vi "patientTrashtListView.vi"() -> ()   [LabVIEW 2019]
uses:
  03_Home/controller/logoutBtn.ctl
  03_Home/controller/exitBtn.ctl
  <vilib>/Utility/miscctls.llb/LVPointTypeDef.ctl
  subVI/patients_state.ctl
  03_Home/controller/pannelState.ctl
  globalValue.vi
panel:
  in  "btnGroup":T1
  in  "backPage":bool
  out "x-y*floor(x/y)":i32
  out "totalCount":string
  out "totalPage":i8
  out "crrentPage":i8
  in  "leftBtn":bool
  in  "rightBtn":bool
  out "patientList":i32(listbox)
  in  "searchBtn":bool
  in  "searchForm":string
  in  "Help Button":bool
  in  "LogOut Button":T2
  in  "Exit Button":T3
  out "userNm":string
  # "/"
  # "|"
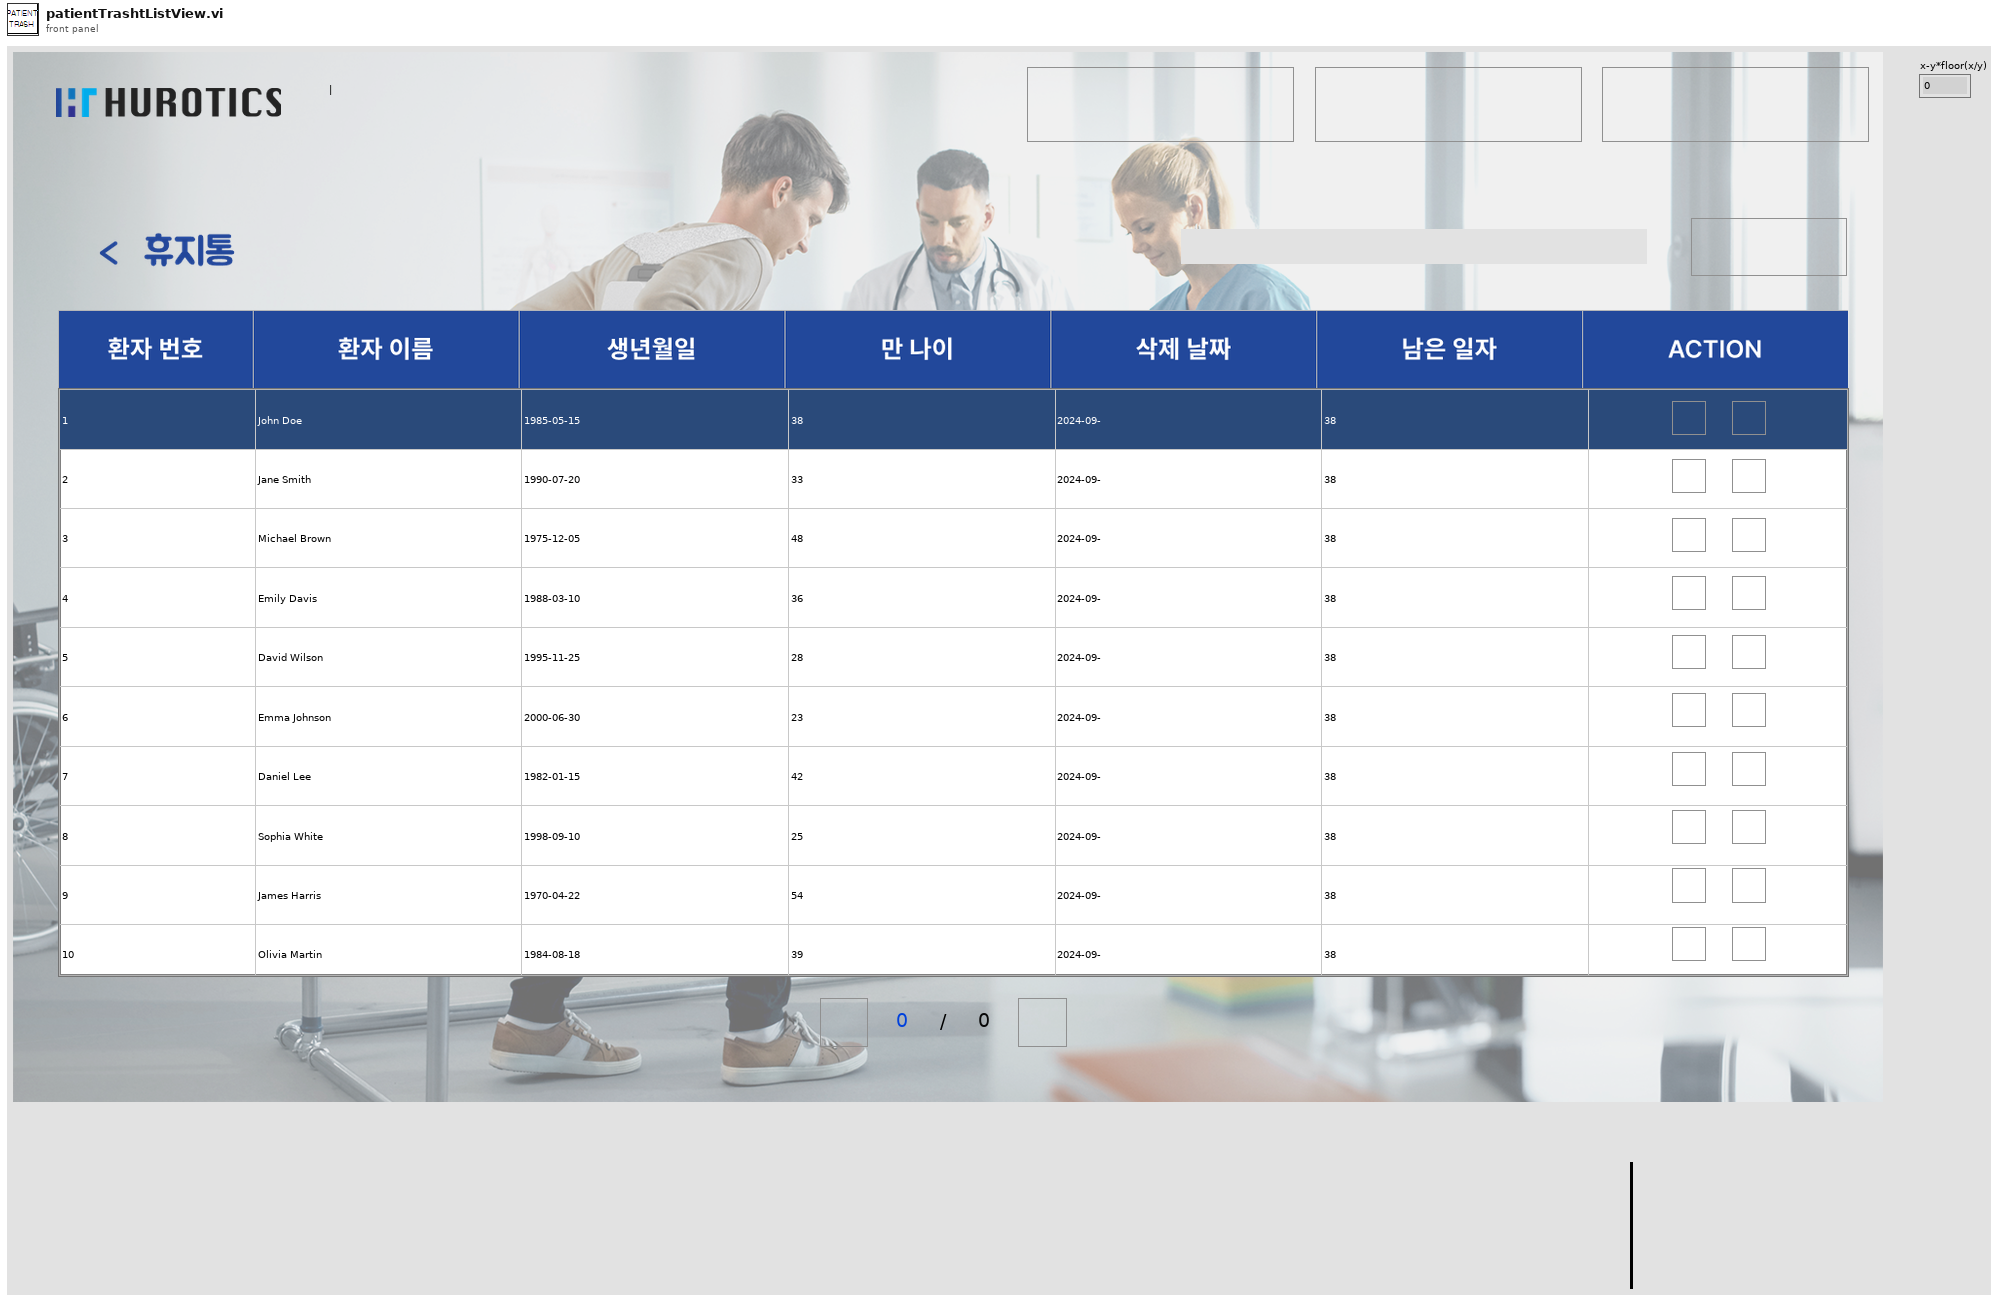
[diagram p1: front panel]
types:
  T1 = cluster{"updateBtn":bool, "deleteBtn":bool, "updateBtn 2":bool, "deleteBtn 2":bool, "updateBtn 3":bool, "deleteBtn 3":bool, "updateBtn 4":bool, "deleteBtn 4":bool, "updateBtn 5":bool, "deleteBtn 5":bool, "updateBtn 6":bool, "deleteBtn 6":bool, "updateBtn 7":bool, "deleteBtn 7":bool, "updateBtn 8":bool, "deleteBtn 8":bool, "updateBtn 9":bool, "deleteBtn 9":bool, "updateBtn 10":bool, "deleteBtn 10":bool}
  T2 = typedef "logoutBtn.ctl" = bool
  T3 = typedef "exitBtn.ctl" = bool
  T4 = typedef "LVPointTypeDef.ctl" = cluster{"Horizontal":i16, "Vertical":i16}
  T5 = enum16{"connection", "create", "getReadList", "getRead", "getCount", "update", "delete", "close"}
  T6 = typedef "patients_state.ctl" = enum16{"connection", "create", "getReadList", "getRead", "getCount", "update", "delete", "trash", "restore", "close"}
  T7 = enum8{"Enabled", "Disabled", "Disabled and Grayed Out"}
  T8 = typedef "pannelState.ctl" = enum16{"Init", "LogIn", "SignUpView", "Home", "Management_patientList", "Management_patientTrashtList", "Management_patientCreate", "Management_patientUpdate", "Management_patientTraining", "Management_patientTrainingDetail", "H-MEDI PatientList", "H-MEDI HardwareCtl", "Adjust", "FineTuning", "UserList", "UserDetail", "Exit"}
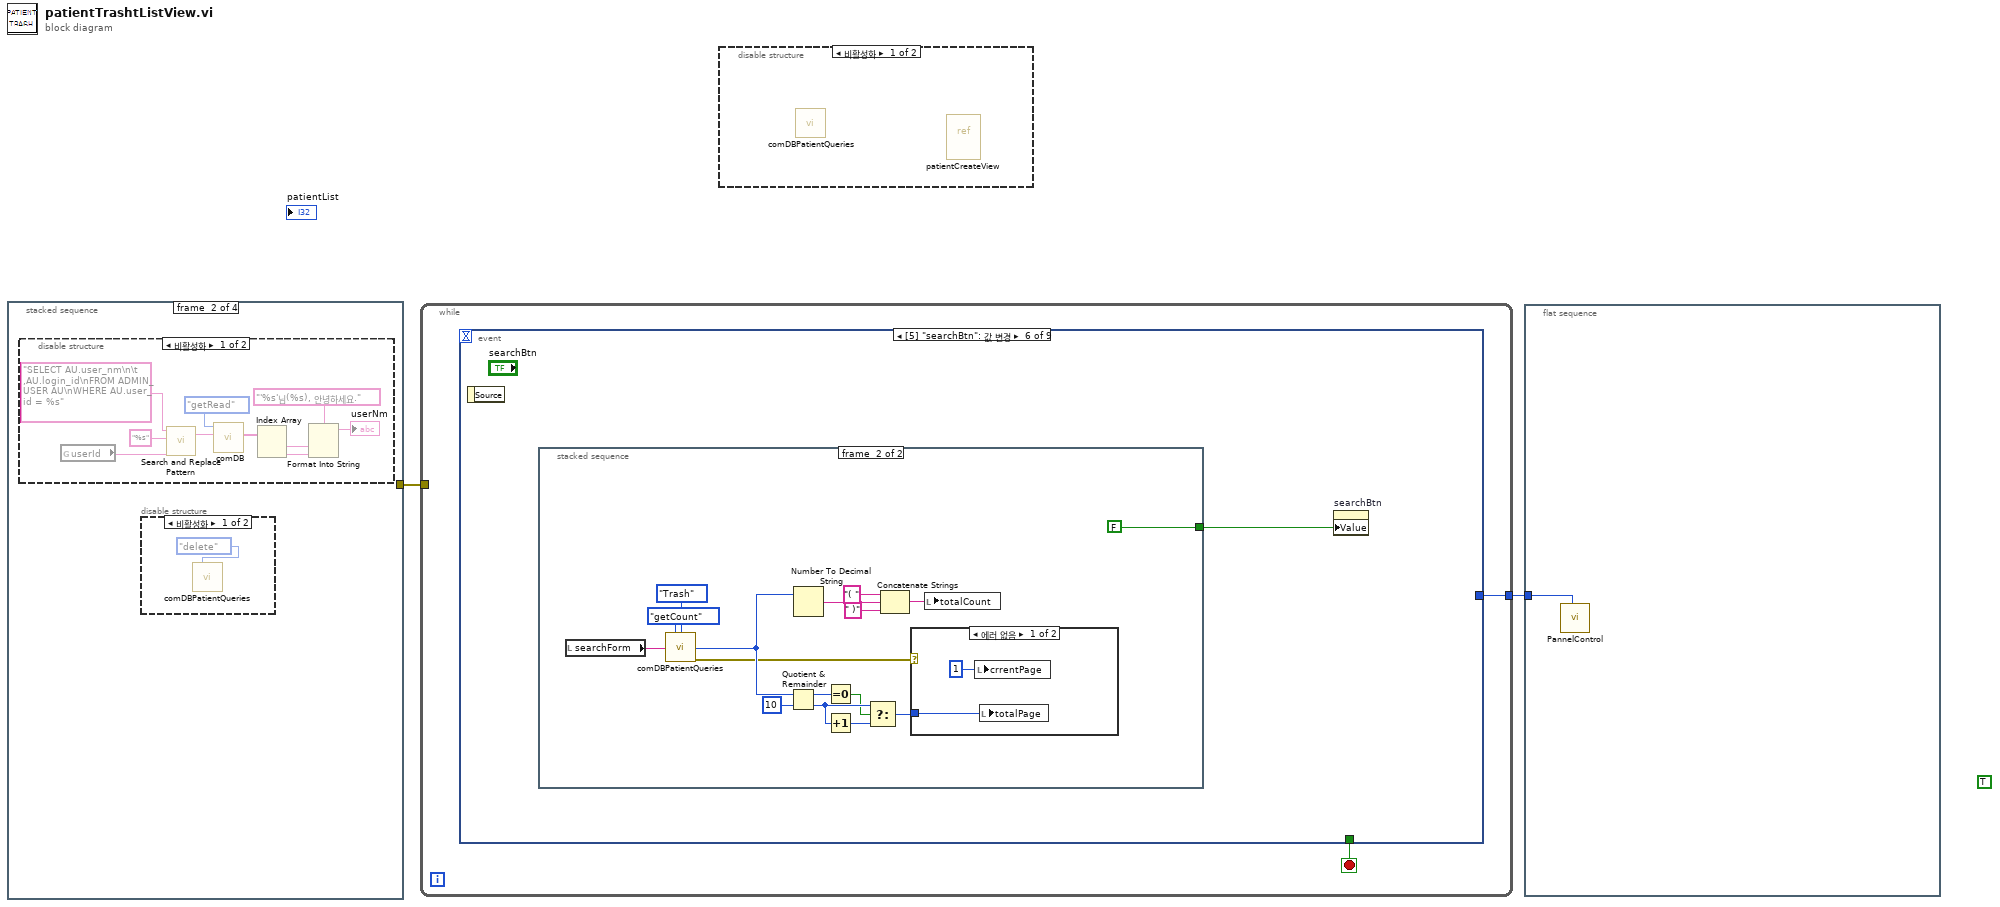
[diagram p0: block diagram]
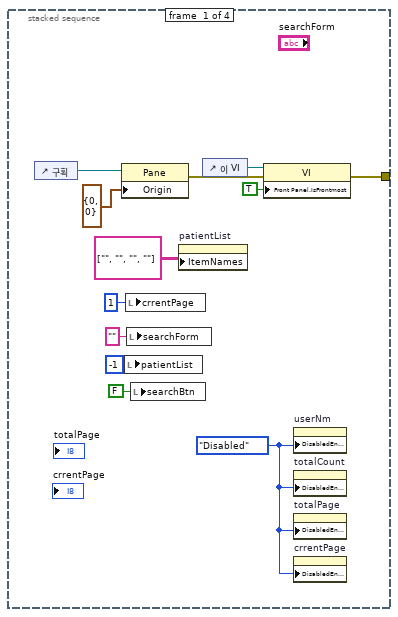
[diagram p3: hidden frame]
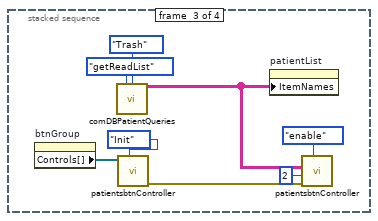
[diagram p6: hidden frame]
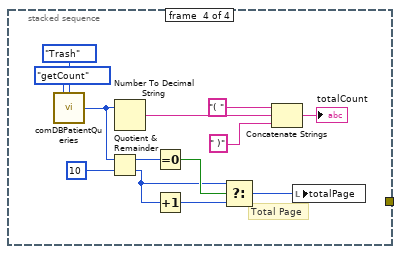
[diagram p7: hidden frame]
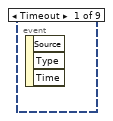
[diagram p8: hidden frame]
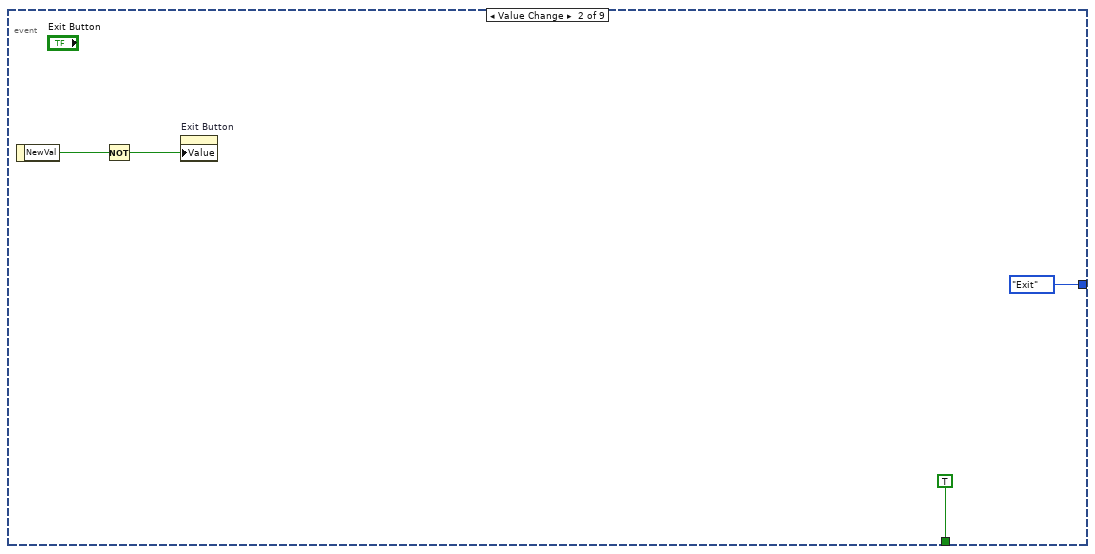
[diagram p9: hidden frame]
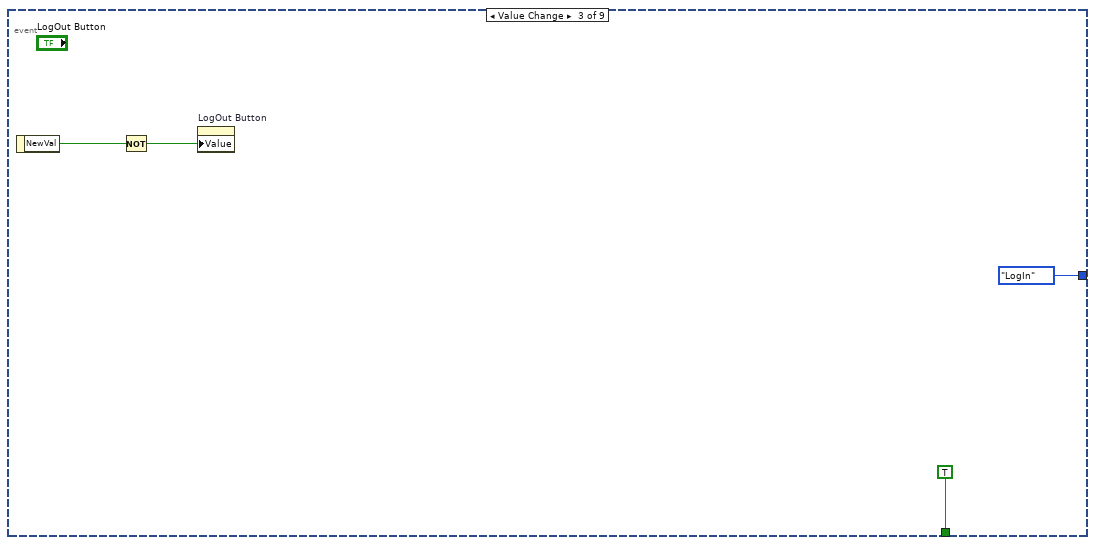
[diagram p10: hidden frame]
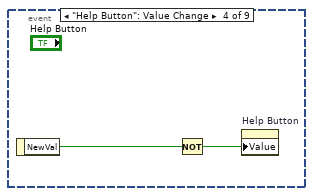
[diagram p11: hidden frame]
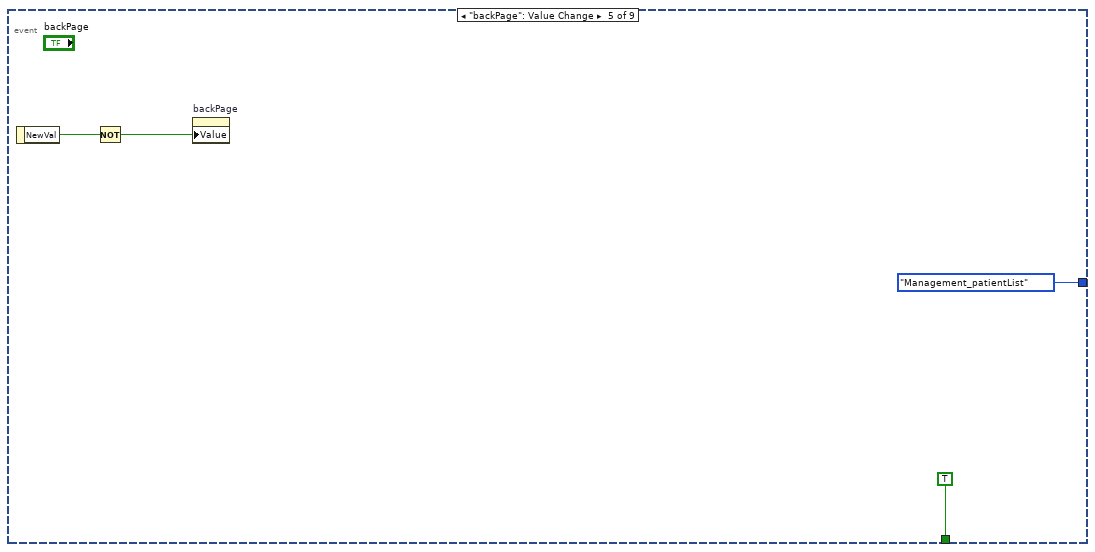
[diagram p12: hidden frame]
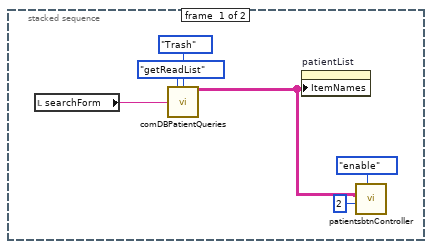
[diagram p13: hidden frame]
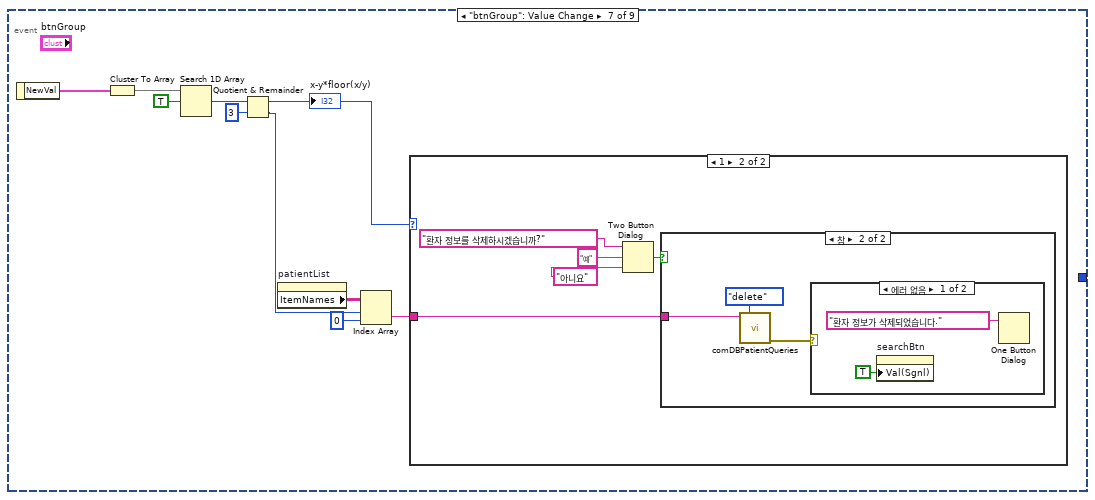
[diagram p15: hidden frame]
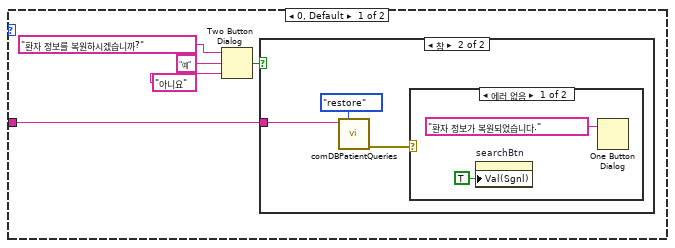
[diagram p16: hidden frame]
diagram:
  (unwired) TRUE
  n1 = stacked-sequence {
    tunnel: [w5 _ _ _] -> w2
    frame #0 {
      w4 = T7."Disabled" ("비활성화")
      n2 = control-ref of="구획"() -> (w12:refnum<vi>)
      n3 = property class="Pane"(reference=w12, "Origin"=T4 {"Horizontal"=0, "Vertical"=0} ("원점")) -> (error out=w10:errorcluster)  [unwired: 1 in, 1 out]
      n4 = local write "patientList"(-1 ("userList")) -> ()
      n5 = local write "crrentPage"(i8 1 ("crrentPage")) -> ()
      n6 = local write "searchForm"("" ("searchForm")) -> ()
      n7 = local write "searchBtn"(FALSE ("searchBtn")) -> ()
      n8 = property on="patientList" class="MCListbox (엄격한)"("ItemNames"=string[][] [["", ""], ["", ""]]) -> ()  [unwired: 2 in, 2 out]
      n9 = control-ref of="이 VI"() -> (w14:refnum<vi>)
      n10 = property class="VI"(reference=w14, error in=w10, "Front Panel.IsFrontmost"=TRUE ("프런트패널 윈도우:맨 앞으로")) -> (error out=w5:errorcluster)  [unwired: 1 out]
      n11 = property on="userNm" class="Str"("DisabledEnum"=w4) -> ()  [unwired: 2 in, 2 out]
      n12 = property on="totalCount" class="Str"("DisabledEnum"=w4) -> ()  [unwired: 2 in, 2 out]
      n13 = property on="totalPage" class="DigNum (엄격한)"("DisabledEnum"=w4) -> ()  [unwired: 2 in, 2 out]
      n14 = property on="crrentPage" class="DigNum (엄격한)"("DisabledEnum"=w4) -> ()  [unwired: 2 in, 2 out]
    }
    frame #1 {
      n15 = disable-structure shown="비활성화" {
        frame Disabled {
          n16 = global read "globalValue.vi" "userId"() -> (w15:string)
          n17 = call <vilib>:"Search and Replace Pattern.vi"("string"="SELECT AU.user_nm\n\t         ,AU.login_id\nFROM ADMIN_USER AU\nWHERE AU.user_id = %s" ("Query"), "regular expression (\"\")"="%s" ("regular expression (\"\")"), "replace string (\"\")"=w15) -> ("result string"=w17:string)  [unwired: 2 in, 1 out]
          n18 = call "comDB.vi"("Query"=w17, "State"=T5."getRead") -> ("result1DArray"=w22:string[])  [unwired: 5 in, 3 out]
          n19 = Index Array(array=w22) -> (element #1=w21:string, element #2=w20:string)  [unwired: 2 in]
          n20 = Format Into String(format string="'%s'님(%s), 안녕하세요." ("문자열"), w21, w20) -> (resulting string=→"userNm":string)  [unwired: 2 in, 1 out]
        }
        frame Enabled {
        }
      }
      n21 = disable-structure shown="비활성화" {
        frame Disabled {
          n22 = call "comDBPatientQueries.vi"("State"=patients_state."delete") -> ()  [unwired: 11 in, 4 out]
        }
        frame Enabled {
        }
      }
    }
    frame #2 {
      n23 = property on="btnGroup" class="Clust"() -> ("Controls[]"=w27:refnum<vi>[])  [unwired: 2 in, 2 out]
      n24 = call "comDBPatientQueries.vi"("State"=patients_state."getReadList", "select"=enum16{"Default", "Trash", "Training"}."Trash") -> ("resultList"=w29:string[][])  [unwired: 10 in, 3 out]
      n25 = call "patientsbtnController.vi"("state"=enum16{"Init", "disable", "enable"}."Init", "Controls[]"=w27) -> ("error out"=w30:errorcluster)  [unwired: 9 in]
      n26 = property on="patientList" class="MCListbox (엄격한)"("ItemNames"=w29) -> ()  [unwired: 2 in, 2 out]
      n27 = call "patientsbtnController.vi"("state"=enum16{"Init", "disable", "enable"}."enable", "error in (no error)"=w30, "버튼개수"=2, "2dArray"=w29) -> ()  [unwired: 7 in, 1 out]
    }
    frame #3 {
      # "Total Page"
      n28 = call "comDBPatientQueries.vi"("State"=patients_state."getCount", "select"=enum16{"Default", "Trash", "Training"}."Trash") -> ("count"=w35:i64)  [unwired: 10 in, 3 out]
      n29 = Quotient & Remainder(x=w35, y=i64 10) -> (x-y*floor(x/y)=w38:i64, floor(x/y)=w37:i64)
      n30 = Number To Decimal String(number=w35) -> (decimal integer string=w44:string)  [unwired: 1 in]
      n31 = Equal To 0?(x=w38) -> (x = 0?=w39:bool)
      n32 = Increment(x=w37) -> (x+1=w41:i64)
      n33 = Select(t=w37, s=w39, f=w41) -> (s? t:f=w40:i64)
      n34 = Concatenate Strings("( ", w44, " )") -> (→"totalCount":string)
      n35 = local write "totalPage"(w40) -> ()
    }
  }
  n36 = while {
    tunnel: w2 -> [_]
    tunnel: [w47] -> w1
    stop <- w48 stop-if-true
    n37 = event shown="[5] \"searchBtn\": 값 변경" {
      selector: _ -> [_ _ _ _ _ _ _ _ _]
      dyn-events: _ -> [_ _ _ _ _ _ _ _ _]
      timeout: _ -> [_ _ _ _ _ _ _ _ _]
      tunnel: [_ TRUE TRUE _ TRUE _ _ _ _] -> w48
      tunnel: [_ pannelState."Exit" ("State") pannelState."LogIn" ("State") _ pannelState."Management_patientList" ("State") _ _ _ _] -> w47
      event Timeout {
        n38 = event-data() -> ()  [unwired: 1 in, 3 out]
      }
      event Value Change {
        n39 = event-data() -> ("NewVal"=w50:T3)  [unwired: 1 in]
        n40 = Not(x=w50) -> (.not. x?=w49:T3)
        n41 = property on="Exit Button" class="Bool (엄격한)"("Value"=w49) -> ()  [unwired: 2 in, 2 out]
      }
      event Value Change {
        n42 = event-data() -> ("NewVal"=w56:T2)  [unwired: 1 in]
        n43 = Not(x=w56) -> (.not. x?=w55:T2)
        n44 = property on="LogOut Button" class="Bool (엄격한)"("Value"=w55) -> ()  [unwired: 2 in, 2 out]
      }
      event "Help Button": Value Change {
        n45 = event-data() -> ("NewVal"=w58:bool)  [unwired: 1 in]
        n46 = Not(x=w58) -> (.not. x?=w57:bool)
        n47 = property on="Help Button" class="Bool (엄격한)"("Value"=w57) -> ()  [unwired: 2 in, 2 out]
      }
      event "backPage": Value Change {
        n48 = event-data() -> ("NewVal"=w60:bool)  [unwired: 1 in]
        n49 = Not(x=w60) -> (.not. x?=w59:bool)
        n50 = property on="backPage" class="Bool (엄격한)"("Value"=w59) -> ()  [unwired: 2 in, 2 out]
      }
      event "searchBtn": Value Change {
        n51 = event-data() -> ()  [unwired: 1 in, 1 out]
        n52 = stacked-sequence {
          tunnel: [_ FALSE ("searchBtn")] -> w63
          frame #0 {
            n53 = local read "searchForm"() -> (w67:string)
            n54 = call "comDBPatientQueries.vi"("State"=patients_state."getReadList", "select"=enum16{"Default", "Trash", "Training"}."Trash", "searchForm"=w67) -> ("resultList"=w66:string[][])  [unwired: 9 in, 3 out]
            n55 = property on="patientList" class="MCListbox (엄격한)"("ItemNames"=w66) -> ()  [unwired: 2 in, 2 out]
            n56 = call "patientsbtnController.vi"("state"=enum16{"Init", "disable", "enable"}."enable", "버튼개수"=2, "2dArray"=w66) -> ()  [unwired: 8 in, 1 out]
          }
          frame #1 {
            n57 = local read "searchForm"() -> (w73:string)
            n58 = call "comDBPatientQueries.vi"("State"=patients_state."getCount", "select"=enum16{"Default", "Trash", "Training"}."Trash", "searchForm"=w73) -> ("count"=w72:i64, "error out"=w71:errorcluster)  [unwired: 9 in, 2 out]
            n59 = Quotient & Remainder(x=w72, y=i64 10) -> (x-y*floor(x/y)=w77:i64, floor(x/y)=w78:i64)
            n60 = Number To Decimal String(number=w72) -> (decimal integer string=w82:string)  [unwired: 1 in]
            n61 = Equal To 0?(x=w77) -> (x = 0?=w76:bool)
            n62 = Increment(x=w78) -> (x+1=w80:i64)
            n63 = Select(t=w78, s=w76, f=w80) -> (s? t:f=w79:i64)
            n64 = Concatenate Strings("( ", w82, " )") -> (w83:string)
            n65 = case shown="에러 없음" w71 {
              tunnel: w79 -> [w86 _]
              frame No Error {
                n66 = local write "crrentPage"(i8 1 ("crrentPage")) -> ()
                n67 = local write "totalPage"(w86) -> ()
              }
              frame Error {
              }
            }
            n68 = local write "totalCount"(w83) -> ()
          }
        }
        n69 = property on="searchBtn" class="Bool (엄격한)"("Value"=w63) -> ()  [unwired: 2 in, 2 out]
      }
      event "btnGroup": Value Change {
        n70 = event-data() -> ("NewVal"=w89:T1)  [unwired: 1 in]
        n71 = Cluster To Array(cluster=w89) -> (array=w97:bool[])
        n72 = Search 1D Array(1D array=w97, element=TRUE ("원소")) -> (index of element=w96:i32)  [unwired: 1 in]
        n73 = Quotient & Remainder(x=w96, y=3) -> (x-y*floor(x/y)=w90:i32, floor(x/y)=w91:i32)
        "x-y*floor(x/y)" <- w90
        n74 = property on="patientList" class="MCListbox (엄격한)"() -> ("ItemNames"=w94:string[][])  [unwired: 2 in, 2 out]
        n75 = Index Array(array=w94, index (row)=w91, index (col)=0 ("비활성화된 인덱스 (열)")) -> (element=w92:string)
        n76 = case shown="1" w90 {
          tunnel: w92 -> [w99 w109]
          frame 0, Default {
            n77 = Two Button Dialog(message="환자 정보를 복원하시겠습니까?" ("메시지"), 1:"아니요" ("거짓 버튼 이름(\"취소\")"), 2:"예" ("참 버튼 이름(\"확인\")")) -> (T button?=w98:bool)
            n78 = case shown="참" w98 {
              tunnel: w99 -> [_ w104]
              frame False {
              }
              frame True {
                n79 = call "comDBPatientQueries.vi"("id"=w104, "State"=patients_state."restore") -> ("error out"=w103:errorcluster)  [unwired: 10 in, 3 out]
                n80 = case shown="에러 없음" w103 {
                  frame No Error {
                    n81 = property on="searchBtn" class="Bool (엄격한)"("Val(Sgnl)"=TRUE ("값(신호)")) -> ()  [unwired: 2 in, 2 out]
                    n82 = One Button Dialog(message="환자 정보가 복원되었습니다." ("메시지")) -> ()  [unwired: 1 in, 1 out]
                  }
                  frame Error {
                  }
                }
              }
            }
          }
          frame 1 {
            n83 = Two Button Dialog(message="환자 정보를 삭제하시겠습니까?" ("메시지"), 1:"아니요" ("거짓 버튼 이름(\"취소\")"), 2:"예" ("참 버튼 이름(\"확인\")")) -> (T button?=w108:bool)
            n84 = case shown="참" w108 {
              tunnel: w109 -> [_ w114]
              frame False {
              }
              frame True {
                n85 = call "comDBPatientQueries.vi"("id"=w114, "State"=patients_state."delete") -> ("error out"=w113:errorcluster)  [unwired: 10 in, 3 out]
                n86 = case shown="에러 없음" w113 {
                  frame No Error {
                    n87 = property on="searchBtn" class="Bool (엄격한)"("Val(Sgnl)"=TRUE ("값(신호)")) -> ()  [unwired: 2 in, 2 out]
                    n88 = One Button Dialog(message="환자 정보가 삭제되었습니다." ("메시지")) -> ()  [unwired: 1 in, 1 out]
                  }
                  frame Error {
                  }
                }
              }
            }
          }
        }
      }
      event "leftBtn": Value Change {
        n89 = event-data() -> ()  [unwired: 1 in, 1 out]
        n90 = local read "crrentPage"() -> (w118:i8)
        n91 = Greater?(x=w118, y=1) -> (0:w120:bool)
        n92 = case shown="참" w120 {
          frame False {
          }
          frame True {
            n93 = local read "searchForm"() -> (w125:string)
            n94 = local read "crrentPage"() -> (w128:i8)
            n95 = Decrement(x=w128) -> (x-1=w127:i8)
            n96 = Number To Decimal String(number=w127) -> (decimal integer string=w124:string)  [unwired: 1 in]
            n97 = call "comDBPatientQueries.vi"("State"=patients_state."getReadList", "select"=enum16{"Default", "Trash", "Training"}."Trash", "searchForm"=w125, "crrentPage"=w124) -> ("resultList"=w122:string[][], "error out"=w123:errorcluster)  [unwired: 8 in, 2 out]
            n98 = property on="patientList" class="MCListbox (엄격한)"("ItemNames"=w122) -> ()  [unwired: 2 in, 2 out]
            n99 = case shown="에러 없음" w123 {
              tunnel: w127 -> [w132 _]
              tunnel: w122 -> [w130 _]
              frame No Error {
                n100 = local write "crrentPage"(w132) -> ()
                n101 = call "patientsbtnController.vi"("state"=enum16{"Init", "disable", "enable"}."enable", "버튼개수"=2, "2dArray"=w130) -> ()  [unwired: 8 in, 1 out]
              }
              frame Error {
              }
            }
          }
        }
      }
      event "rightBtn": Value Change {
        n102 = event-data() -> ()  [unwired: 1 in, 1 out]
        n103 = local read "crrentPage"() -> (w135:i8)
        n104 = local read "totalPage"() -> (w134:i8)
        n105 = Less?(x=w135, y=w134) -> (x < y?=w133:bool)
        n106 = case shown="참" w133 {
          frame False {
          }
          frame True {
            n107 = local read "searchForm"() -> (w140:string)
            n108 = local read "crrentPage"() -> (w143:i8)
            n109 = Increment(x=w143) -> (x+1=w142:i8)
            n110 = Number To Decimal String(number=w142) -> (decimal integer string=w139:string)  [unwired: 1 in]
            n111 = call "comDBPatientQueries.vi"("State"=patients_state."getReadList", "select"=enum16{"Default", "Trash", "Training"}."Trash", "searchForm"=w140, "crrentPage"=w139) -> ("resultList"=w137:string[][], "error out"=w138:errorcluster)  [unwired: 8 in, 2 out]
            n112 = property on="patientList" class="MCListbox (엄격한)"("ItemNames"=w137) -> ()  [unwired: 2 in, 2 out]
            n113 = case shown="에러 없음" w138 {
              tunnel: w142 -> [w147 _]
              tunnel: w137 -> [w145 _]
              frame No Error {
                n114 = local write "crrentPage"(w147) -> ()
                n115 = call "patientsbtnController.vi"("state"=enum16{"Init", "disable", "enable"}."enable", "버튼개수"=2, "2dArray"=w145) -> ()  [unwired: 8 in, 1 out]
              }
              frame Error {
              }
            }
          }
        }
      }
    }
  }
  n116 = disable-structure shown="비활성화" {
    frame Disabled {
      n117 = call "comDBPatientQueries.vi"() -> ()  [unwired: 12 in, 4 out]
      n118 = vi-ref "patientCreateView.vi"() -> ()  [unwired: 1 out]
    }
    frame Enabled {
    }
  }
  n119 = flat-sequence {
    tunnel: w1 -> [w148]
    frame #0 {
      n120 = call "PannelControl.vi"("State"=w148) -> ()  [unwired: 10 in, 1 out]
    }
  }
